vi "Query.vi"(6 "timeout in ms (5000)":i32=5000, 8 "error in (no error)":errorcluster, 10 "Message":refnum<class "MSG.lvclass">, 11 "MSR Parent":refnum<class "Send.lvclass">) -> (0 "error out":errorcluster, 2 "Reply":refnum<class "MSG.lvclass">, 3 "MSR Parent":refnum<class "Send.lvclass">)   [LabVIEW 2011, in "Messenging.lvlib" / "Send.lvclass"]
uses:
  Send.lvclass
  QueueMessenger/QueueMessenger.lvclass
  TextVarientMessage/MSG.lvclass
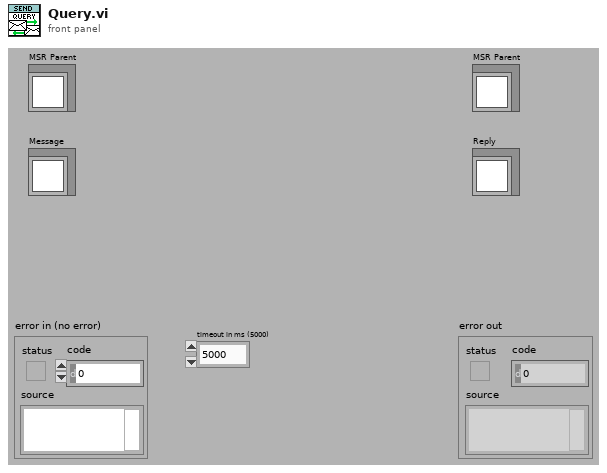
[diagram p1: front panel]
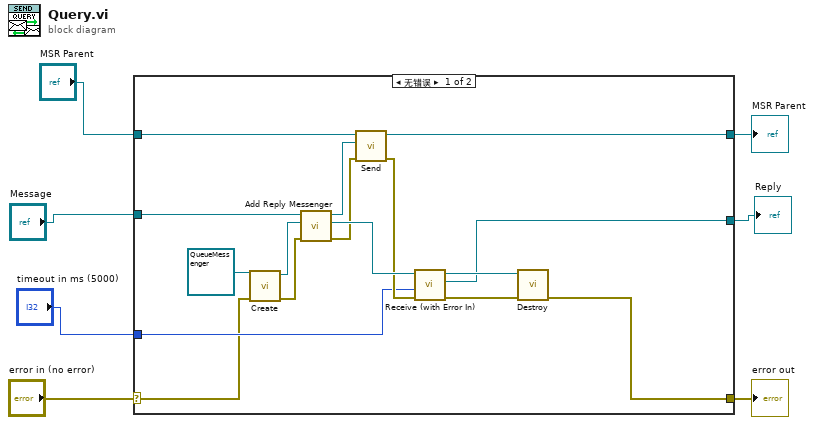
[diagram p0: block diagram]
diagram:
  n1 = case shown="无错误" "error in (no error)" {
    selector: "error in (no error)" -> [w9 w25]
    tunnel: [w8 w25] -> w6
    tunnel: [w15 w24] -> w1
    tunnel: "MSR Parent" -> [w16 w24]
    tunnel: "Message" -> [w17 _]
    tunnel: "timeout in ms (5000)" -> [w11 _]
    tunnel: [w10 _] -> w3
    frame No Error {
      n2 = call-dynamic "Create.vi"("error in (no error)"=w9, "QueueMessenger in"=refnum<class "QueueMessenger.lvclass"> refnum ("QueueMessenger.lvclass")) -> ("error out"=w19:errorcluster, "QueueMessenger out"=w22:refnum<class "QueueMessenger.lvclass">)  [unwired: 8 out]
      n3 = call "Add Reply Messenger.vi"("error in (no error)"=w19, "Reply to..."=w22, "Message"=w17) -> ("error out"=w13:errorcluster, "Reply to..."=w23:refnum<class "QueueMessenger.lvclass">, "Message"=w14:refnum<class "MSG.lvclass">)  [unwired: 6 out]
      n4 = call-dynamic "Send.vi"("error in (no error)"=w13, "Message"=w14, "MSR Parent in"=w16) -> ("error out"=w12:errorcluster, "MSR Parent out"=w15:refnum<class "Send.lvclass">)  [unwired: 7 out]
      n5 = call-dynamic "Receive (with Error In).vi"("error in (no error)"=w12, "timeout in ms (5000)"=w11, "MGR in"=w23) -> ("error out"=w21:errorcluster, "Message"=w10:refnum<class "MSG.lvclass">, "MGR out"=w20:refnum<class "QueueMessenger.lvclass">)  [unwired: 6 out]
      n6 = call-dynamic "Destroy.vi"("error in (no error)"=w21, "QueueMessenger in"=w20) -> ("error out"=w8:errorcluster)  [unwired: 9 out]
    }
    frame Error {
    }
  }
  "error out" <- w6
  "Reply" <- w3
  "MSR Parent" <- w1
